vi "Get Motion Controller.vi"(8 "error in (no error)":errorcluster, 9 "Path":path, 10 "Section":string, 11 "Create Fine Class in":refnum<class "Create Fine Class.lvclass">) -> (0 "error out":errorcluster, 2 "iMotion Controller.lvclass":refnum<class "iMotion Controller.lvclass">, 3 "Create Fine Class out":refnum<class "Create Fine Class.lvclass">)   [LabVIEW 2022 SP3, in "Create Fine Class.lvclass"]
uses:
  Create Fine Class.lvclass
  Motion Controller/FINE SIM Motion Axis.lvclass
  iMotion Controller/iMotion Controller.lvclass
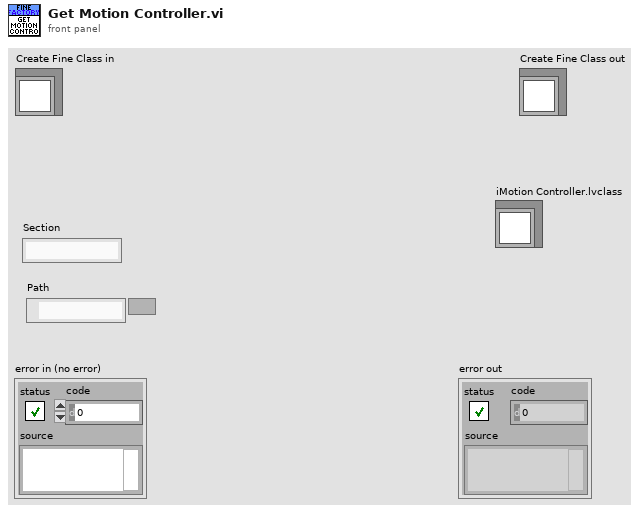
[diagram p1: front panel]
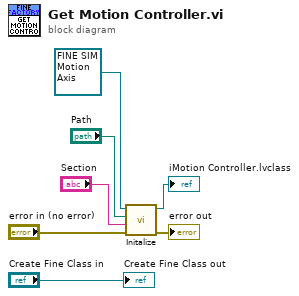
[diagram p0: block diagram]
diagram:
  n1 = call-dynamic "Initalize.vi"("error in (no error)"="error in (no error)", "Section"="Section", "Config Path"="Path", "Motion Controller in"=refnum<class "FINE SIM Motion Axis.lvclass"> refnum ("FINE SIM Motion Axis.lvclass")) -> ("error out"=→"error out":errorcluster, "Motion Controller out"=→"iMotion Controller.lvclass":refnum<class "FINE SIM Motion Axis.lvclass">)  [unwired: 6 in]
  "Create Fine Class out" <- "Create Fine Class in"
